vi "ANC300_Step.vi"(0 "ANC300 Communication Port In":refnum<visa-resource-name>, 1 "connection ID in":refnum<k5>, 2 "Axis":u8(ring)=1 items=["1"=1, "2"=2, "3"=3, "4"=4, "5"=5, "6"=0], 3 "stepping direction":bool=TRUE, 4 "number of steps [0=cont.]":i32=100, 5 "error in":T1, 6 "wait for last step":bool=TRUE, 7 "Time to wait [ms]":u32=200) -> (12 "command string":string, 13 "data out":string, 14 "ANC300 Communication Port Out":refnum<visa-resource-name>, 15 "connection ID out":refnum<k5>, 18 "transfer ok":bool, 19 "error out":T1)   [LabVIEW 2023]
panel:
  out "resulting string":string
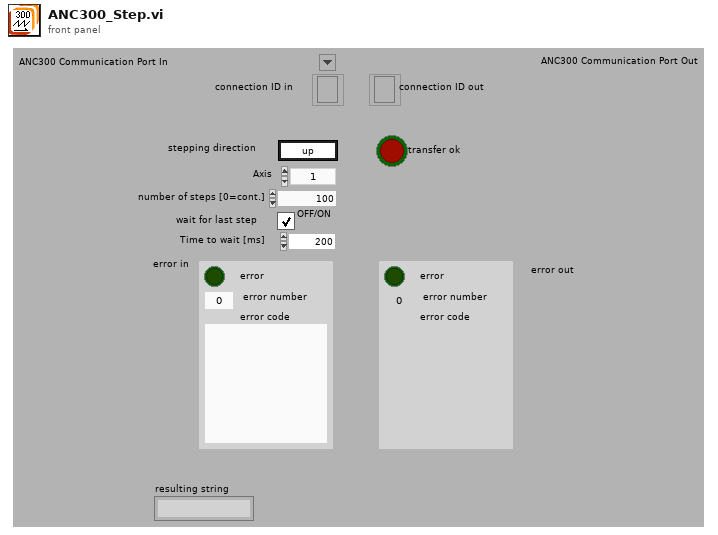
[diagram p1: front panel]
types:
  T1 = cluster{"error ":bool, "error number":i32, "error code":string}
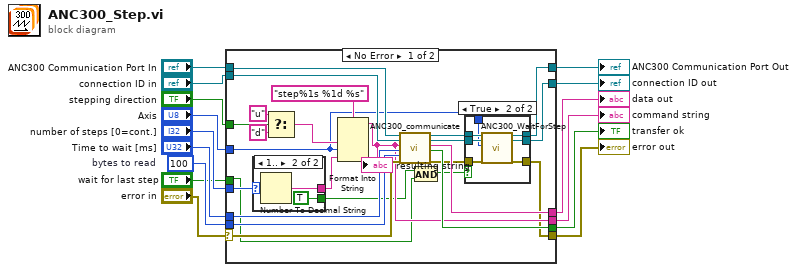
[diagram p0: block diagram]
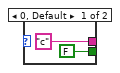
[diagram p3: hidden frame]
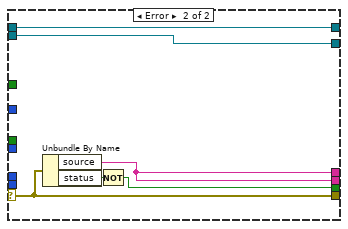
[diagram p4: hidden frame]
diagram:
  w11 = 100  # bytes to read
  n1 = case shown="No Error" "error in" {
    selector: "error in" -> [w36 w59]
    tunnel: "Axis" -> [w19 _]
    tunnel: "stepping direction" -> [w30 _]
    tunnel: "ANC300 Communication Port In" -> [w40 w61]
    tunnel: "connection ID in" -> [w39 w60]
    tunnel: "Time to wait [ms]" -> [w38 _]
    tunnel: w11 -> [w37 _]
    tunnel: [w24 w59] -> w5
    tunnel: [w21 w61] -> w9
    tunnel: [w20 w60] -> w8
    tunnel: [w35 w57] -> w4
    tunnel: [w29 w56] -> w7
    tunnel: [w34 w56] -> w6
    tunnel: "number of steps [0=cont.]" -> [w32 _]
    tunnel: "wait for last step" -> [w16 _]
    frame No Error {
      n2 = case shown="1.." w32 {
        selector: w32 -> [_ w55]
        tunnel: ["c" w54] -> w27
        tunnel: [FALSE TRUE] -> w17
        frame 0, Default {
        }
        frame 1.. {
          n3 = Number To Decimal String(number=w55) -> (decimal integer string=w54:string)  [unwired: 1 in]
        }
      }
      n4 = Select(t="u", s=w30, f="d") -> (s? t:f=w28:string)
      n5 = Format Into String(format string="step%1s %1d %s", w28, w19, w27) -> (resulting string=w29:string)  [unwired: 2 in, 1 out]
      "resulting string" <- w29
      n6 = call "ANC300_communicate.vi"("ANC300 Communication Port In"=w40, "connection ID in"=w39, "commando string"=w29, "Time to wait [ms]"=w38, "bytes to read"=w37, "error in"=w36) -> ("ANC300 Communication Port Out"=w23:refnum<visa-resource-name>, "connection ID out"=w22:refnum<k5>, "read data"=w34:string, "transfer ok"=w35:bool, "error out"=w25:T1)  [unwired: 9 in]
      n7 = And(x=w17, y=w16) -> (x .and. y?=w18:bool)
      n8 = case shown="True" w18 {
        tunnel: w25 -> [w42 w50]
        tunnel: [w42 w49] -> w24
        tunnel: w23 -> [w43 w48]
        tunnel: w22 -> [w41 w47]
        tunnel: [w43 w46] -> w21
        tunnel: [w41 w45] -> w20
        tunnel: w19 -> [_ w44]
        frame False {
        }
        frame True {
          n9 = call "ANC300_WaitForStep.vi"("ANC300 Communication Port In"=w48, "connection ID in"=w47, "Axis"=w44, "error in"=w50) -> ("ANC300 Communication Port Out"=w46:refnum<visa-resource-name>, "connection ID out"=w45:refnum<k5>, "error out"=w49:T1)  [unwired: 10 in, 3 out]
        }
      }
    }
    frame Error {
      n10 = Unbundle By Name(w59) -> ("source"=w56:string, "status"=w58:bool)
      n11 = Not(x=w58) -> (.not. x?=w57:bool)
    }
  }
  "data out" <- w6
  "connection ID out" <- w8
  "error out" <- w5
  "command string" <- w7
  "transfer ok" <- w4
  "ANC300 Communication Port Out" <- w9
